vi "FTW-ERR-StatusException.vi"(1 "error to check":errorcluster) -> (0 "Exception":T1)   [LabVIEW 2012]
uses:
  FTW-ERR-ExceptionType.ctl
panel:
  # "Inputs"
  # "Outputs"
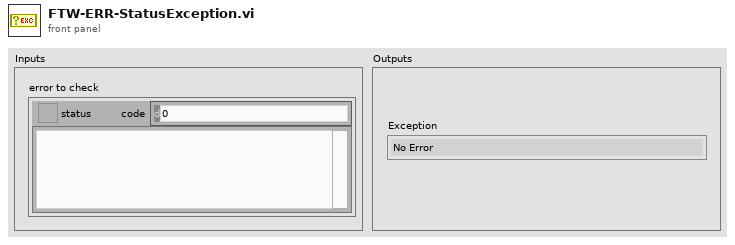
[diagram p1: front panel]
types:
  T1 = typedef "FTW-ERR-ExceptionType.ctl" = enum16{"No Error", "Error", "Warning"}
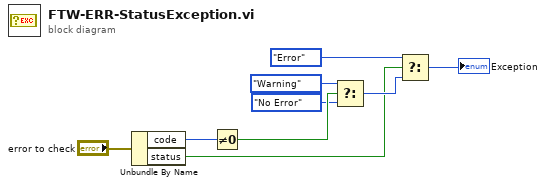
[diagram p0: block diagram]
diagram:
  n1 = Unbundle By Name("error to check") -> ("code"=w9:i32, "status"=w1:bool)
  n2 = Not Equal To 0?(x=w9) -> (x != 0?=w7:bool)
  n3 = Select(t=FTW-ERR-ExceptionType."Warning" ("Exception"), s=w7, f=FTW-ERR-ExceptionType."No Error" ("Exception")) -> (s? t:f=w6:T1)
  n4 = Select(t=FTW-ERR-ExceptionType."Error" ("Exception"), s=w1, f=w6) -> (s? t:f=→"Exception":T1)
